vi "One Dynamic Input One Dynamic Output.vi"(8 "error in (no error)":errorcluster, 11 "Class Alpha in":refnum<class "Class Alpha.lvclass">) -> (0 "error out":errorcluster, 3 "Class Alpha out":refnum<class "Class Alpha.lvclass">)   [LabVIEW 2023, in "Class Alpha.lvclass"]
doc: "This VI is an example of a dynamic member VI with one dynamic output terminal. It modifies the input object."
uses:
  Class Alpha.lvclass
  Class Alpha.lvclass/Class Alpha.ctl
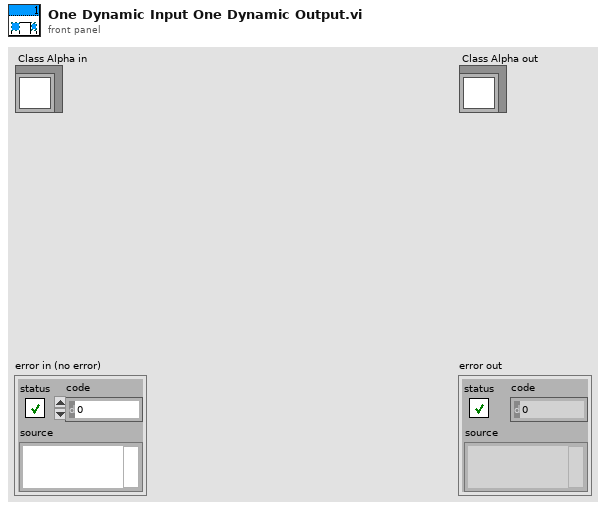
[diagram p1: front panel]
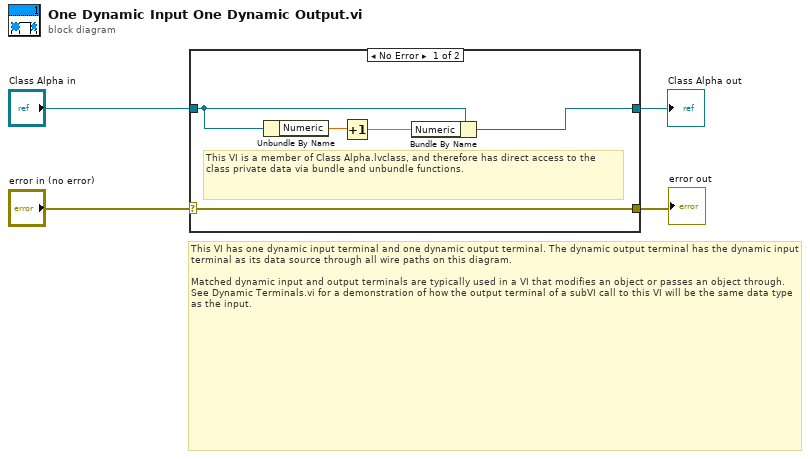
[diagram p0: block diagram]
diagram:
  # "This VI has one dynamic input terminal and one dynamic output terminal. The dynamic output terminal has the dynamic input terminal as its data source through all wire paths on this diagram.\n\nMatched dynamic input and output terminals are typically used in a VI that modifies an object or passes an object through. See Dynamic Terminals.vi for a demonstration of how the output terminal of a subVI call to this VI will be the same data type as the input."
  n1 = case shown="No Error" "error in (no error)" {
    selector: "error in (no error)" -> [w9 w11]
    tunnel: [w9 w11] -> w3
    tunnel: [w5 w10] -> w1
    tunnel: "Class Alpha in" -> [w6 w10]
    frame No Error {
      # "This VI is a member of Class Alpha.lvclass, and therefore has direct access to the class private data via bundle and unbundle functions."
      n2 = Unbundle By Name(w6) -> ("Numeric"=w8:dbl)
      n3 = Increment(x=w8) -> (x+1=w7:dbl)
      n4 = Bundle By Name(cluster=w6, "Numeric"=w7) -> (w5:refnum<class "Class Alpha.lvclass">)
    }
    frame Error {
    }
  }
  "error out" <- w3
  "Class Alpha out" <- w1
